vi "GaussianFindPeak.vi"(0 "Input XY":T5, 2 "method":T4 items=["Least Square", "Least Absolute Residual", "Bisquare"]) -> (3 "Gauss Result":T2, 4 "Origin+Fit":T1(array[cluster]))   [LabVIEW 2020]
uses:
  <vilib>/Analysis/6fits.llb/Curve Fitting Criteria.ctl
  <vilib>/Analysis/NI_AALPro.lvlib
panel:
  in  "parameter bounds":T3={"amp min"=0.0, "amp max"=inf, "center min"=-inf, "center max"=inf, "deviation min"=-inf, "deviation max"=inf, "offset min"=100.0, "offset max"=50000.0}
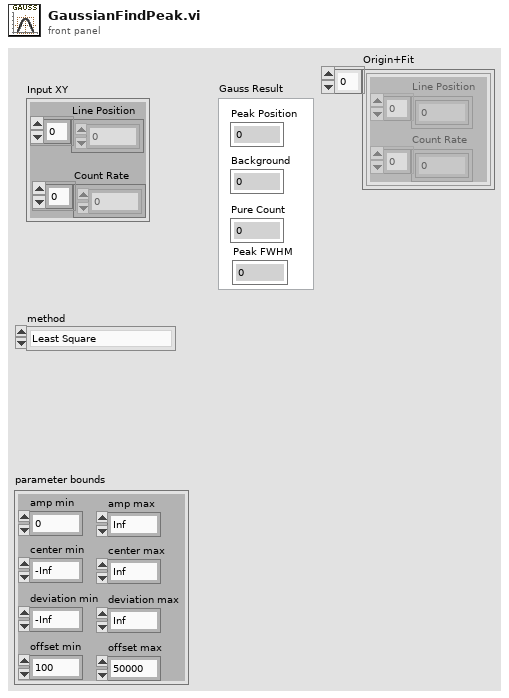
[diagram p1: front panel]
types:
  T1 = cluster{"Line Position":dbl[], "Count Rate":dbl[]}[]
  T2 = cluster{"Peak Position":dbl, "Background":dbl, "Pure Count":dbl, "Peak FWHM":dbl}
  T3 = cluster{"amp min":dbl, "amp max":dbl, "center min":dbl, "center max":dbl, "deviation min":dbl, "deviation max":dbl, "offset min":dbl, "offset max":dbl}
  T4 = typedef "NI_AALPro.lvlib/Curve Fitting Criteria.ctl" = u16
  T5 = cluster{"Line Position":dbl[], "Count Rate":dbl[]}
  T6 = cluster{"initial amplitude":dbl, "initial center":dbl, "initial standard deviation":dbl, "offset":dbl}
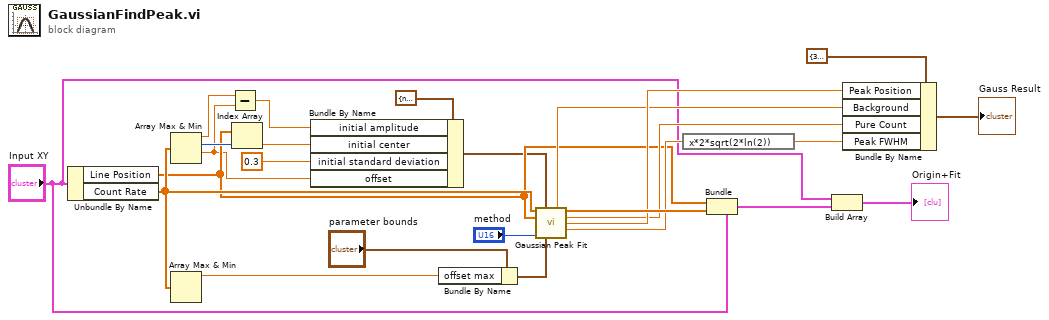
[diagram p0: block diagram]
diagram:
  n1 = Unbundle By Name("Input XY") -> ("Line Position"=w8:dbl[], "Count Rate"=w10:dbl[])
  n2 = Array Max & Min(array=w10) -> (max value=w6:dbl, max index (indices)=w9:i32, min value=w3:dbl)  [unwired: 1 out]
  n3 = Array Max & Min(array=w10) -> (max value=w19:dbl)  [unwired: 3 out]
  n4 = Subtract(x=w6, y=w3) -> (x-y=w5:dbl)
  n5 = Index Array(array=w8, index=w9) -> (element=w7:dbl)
  n6 = Bundle By Name(cluster=T6 {"initial amplitude"=nan, "initial center"=nan, "initial standard deviation"=nan, "offset"=nan} ("initial guess"), "initial amplitude"=w5, "initial center"=w7, "initial standard deviation"=0.3, "offset"=w3) -> (w1:T6)
  n7 = Bundle By Name(cluster="parameter bounds", "offset max"=w19) -> (w18:T3)
  n8 = call <vilib>:"Gaussian Peak Fit.vi"("Y"=w10, "initial guess"=w1, "X"=w8, "method"="method", "parameter bounds"=w18) -> ("offset"=w22:dbl, "Best Gaussian Fit"=w24:dbl[], "amplitude"=w21:dbl, "center"=w23:dbl, "standard deviation"=w15:dbl)  [unwired: 4 in, 2 out]
  n9 = expression code="x*2*sqrt(2*ln(2))"(w15) -> (w14:dbl)
  n10 = Bundle(cluster="Input XY", "Line Position"=w8, "Count Rate"=w24) -> (w12:T5)
  n11 = Build Array("Input XY", w12) -> (→"Origin+Fit":T1)
  n12 = Bundle By Name(cluster=T2 {"Peak Position"=31.987915688519237, "Background"=2498.538860968832, "Pure Count"=10359.489225155847, "Peak FWHM"=10359.489225155847} ("Gauss Result"), "Peak Position"=w23, "Background"=w22, "Pure Count"=w21, "Peak FWHM"=w14) -> (→"Gauss Result":T2)
